vi "Select COM for AutoBaud.vi"(8 "error in (no error)":errorcluster, 9 "Port Name":string, 10 "VI reference (current VI)":refnum<vi>, 11 "VISA resource name 2":refnum<visa-resource-name>) -> (0 "error out":errorcluster, 2 ".not. x?":bool, 3 "VISA resource name out":refnum<visa-resource-name>)   [LabVIEW 2017]
panel:
  out "String":string
  in  "Blank Button":bool
  in  "VISA resource name":refnum<visa-resource-name>
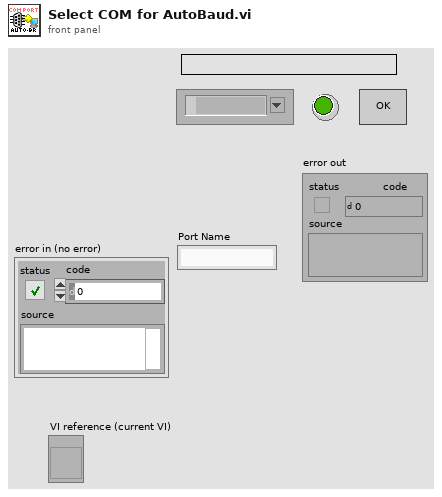
[diagram p1: front panel]
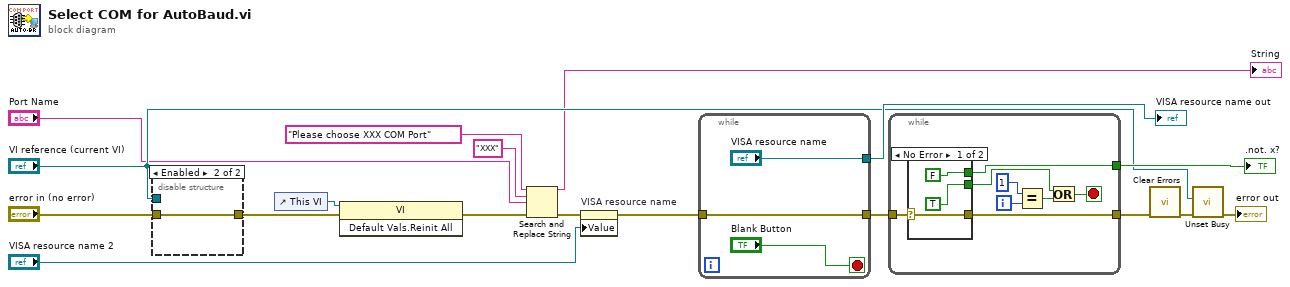
[diagram p0: block diagram]
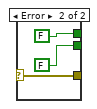
[diagram p2: hidden frame]
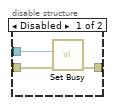
[diagram p3: hidden frame]
diagram:
  n1 = disable-structure shown="Enabled" {
    disable-tunnel: "VI reference (current VI)" -> [w21 _]
    disable-tunnel: "error in (no error)" -> [w20 w22]
    disable-tunnel: [w19 w22] -> w11
    frame Disabled {
      n2 = call <vilib>:"Set Busy.vi"("error in (no error)"=w20, "VI reference (current VI)"=w21) -> ("error out"=w19:errorcluster)  [unwired: 8 in, 1 out]
    }
    frame Enabled {
    }
  }
  n3 = control-ref of="This VI"() -> (w18:refnum<vi>)
  n4 = invoke class="VI" method="Default Vals.Reinit All"(reference=w18, error in=w11) -> (error out=w2:errorcluster)  [unwired: 1 in, 2 out]
  n5 = Search and Replace String(input string="Please choose XXX COM Port", search string="XXX", replace string="Port Name", error in=w2) -> (result string=→"String":string, error out=w1:errorcluster)  [unwired: 4 in, 2 out]
  n6 = property on="VISA resource name" class="VISAName"(error in=w1, "Value"="VISA resource name 2") -> (error out=w10:errorcluster)  [unwired: 1 in, 1 out]
  n7 = while {
    tunnel: ["VISA resource name"] -> w16
    tunnel: w10 -> [w23]
    tunnel: [w23] -> w9
    stop <- "Blank Button" stop-if-true
  }
  "VISA resource name out" <- w16
  n8 = while {
    tunnel: [w32] -> w13
    tunnel: w9 -> [w31]
    tunnel: [w33] -> w15
    i -> [w28]
    stop <- w29 stop-if-true
    n9 = case shown="No Error" w31 {
      selector: w31 -> [w36 w38]
      tunnel: [w36 w38] -> w33
      tunnel: [FALSE FALSE] -> w32
      tunnel: [TRUE FALSE] -> w30
      frame No Error {
      }
      frame Error {
      }
    }
    n10 = Equal?(x=1, y=w28) -> (x = y?=w26:bool)
    n11 = Or(x=w30, y=w26) -> (x .or. y?=w29:bool)
  }
  ".not. x?" <- w13
  n12 = call <vilib>:"Clear Errors.vi"("error in (no error)"=w15) -> ("error out"=w14:errorcluster)  [unwired: 5 in, 1 out]
  n13 = call <vilib>:"Unset Busy.vi"("error in (no error)"=w14, "VI reference (current VI)"="VI reference (current VI)") -> ("error out"=→"error out":errorcluster)  [unwired: 9 in]
